vi "Robot Global Data.vi"() -> ()   [LabVIEW 2015]
doc: "This global VI can contain as many global variables as you need. Place a control on the panel, give it a good name. To read or write to it from a VI, drag the icon to the diagram of that VI. You can also drag from the project. Click on the node to change which global you access. You shouldn't have multiple locations writing to a global or it will cause a race-condition."
uses:
  <vilib>/Rock Robotics/WPI/Camera/WPI_CameraImageSize.ctl
  <vilib>/Rock Robotics/WPI/DriverStation/WPI_DriverStationRobotMode2.ctl
panel:
  in  "THIS CASE":string
  in  "test":enum16{"1 Tote", "1 Bin", "3 Totes"}(ring)
  in  "arcade value":dbl
  in  "reset pot":dbl
  in  "potDistance":dbl
  in  "potValue":dbl
  in  "distance":dbl
  in  "Case":string
  in  "initial gyro":dbl
  in  "Reset gyro":bool
  in  "gyro":dbl
  in  "Reset Encoders":bool
  in  "right encoder":dbl
  in  "left encoder":dbl
  in  "Autonomous Mode":T1(ring)
  in  "bottomSwitch":bool
  in  "topSwitch":bool
  in  "Robot Mode":T2
  in  "image size":T3=enum."320x240"
  in  "Enable Vision":bool
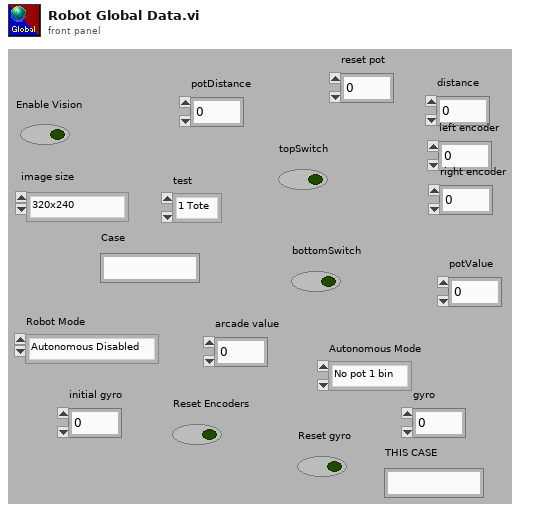
[diagram p1: front panel]
types:
  T1 = enum16{"No pot 1 bin", "3 Tote Spinny", "2 Tote Middle", "1 Bin", "1 Tote", "Drive", "3 Tote"}
  T2 = typedef "WPI_DriverStationRobotMode2.ctl" = enum16{"Autonomous Disabled", "Autonomous Enabled", "Teleop Disabled", "Teleop Enabled", "Disconnected", "Finish", "Test Disabled", "Test Enabled", "Emergency Stopped"}
  T3 = typedef "WPI_CameraImageSize.ctl" = enum16{"640x480", "320x240", "160x120", "Custom"}
diagram:
